vi "Open TCP Connection.vi"(8 "error in (no error)":errorcluster, 10 "timeout ms (60000)":i32, 11 "network address":string) -> (0 "error out":errorcluster, 3 "TCP Network Connection out":refnum<k5>)   [LabVIEW 2019, in "TimingDRV System Explorer.lvlib"]
uses:
  TimingDRV System Explorer.lvlib
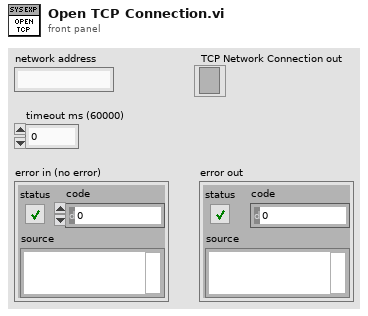
[diagram p1: front panel]
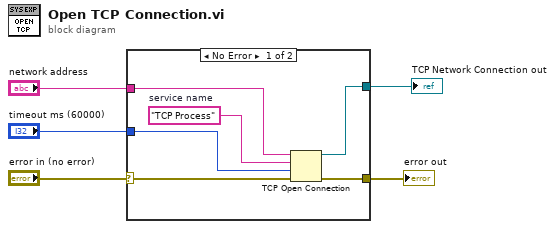
[diagram p0: block diagram]
diagram:
  n1 = case shown="No Error" "error in (no error)" {
    selector: "error in (no error)" -> [w6 w12]
    tunnel: [w11 _] -> w5
    tunnel: [w10 w12] -> w4
    tunnel: "timeout ms (60000)" -> [w9 _]
    tunnel: "network address" -> [w8 _]
    frame No Error {
      w7 = "TCP Process"  # service name
      n2 = TCP Open Connection(address=w8, remote port or service name=w7, timeout ms (60000)=w9, error in (no error)=w6) -> (connection ID=w11:refnum<k5>, error out=w10:errorcluster)  [unwired: 1 in]
    }
    frame Error {
    }
  }
  "TCP Network Connection out" <- w5
  "error out" <- w4
